vi "TreeItem.Get.vi"(8 "error in (no error)":errorcluster, 9 "Tree":T1[](array[typedef]) {"Properties"."Type" items=["K_STRING", "K_BOOL", "K_I32", "K_U32", "K_DOUBLE", "K_U64", "K_VARIANT", "K_DEPENDENTFILE", "K_DEPENDENTNODE", "K_DATASOURCENODE", "K_U16", "K_DBLARR", "K_U32ARR", "K_I32ARR", "K_STRINGARR", "K_DICTIONARY", "K_DICTIONARYARR"]}, 10 "CustomDevice BaseNode Ref":refnum<k24>, 11 "NodeIDUtil Ref":refnum<k24>) -> (0 "error out":errorcluster, 1 "Tree":T1[](array[typedef]) {"Properties"."Type" items=["K_STRING", "K_BOOL", "K_I32", "K_U32", "K_DOUBLE", "K_U64", "K_VARIANT", "K_DEPENDENTFILE", "K_DEPENDENTNODE", "K_DATASOURCENODE", "K_U16", "K_DBLARR", "K_U32ARR", "K_I32ARR", "K_STRINGARR", "K_DICTIONARY", "K_DICTIONARYARR"]}, 2 "CustomDevice BaseNode Ref out":refnum<k24>, 3 "NodeIDUtil Ref out":refnum<k24>)   [LabVIEW 2015, in "System Definition Utilities.lvlib"]
uses:
  System Definition Utilities.lvlib
  _Types/TreeItem.ctl
  _Types/TreeItem.Info.ctl
  <vilib>/NI Veristand/Custom Device API/Custom Device Channel.ctl
  <vilib>/NI Veristand/Custom Device API/Custom Device Channel Type.ctl
  <vilib>/NI Veristand/Custom Device API/Custom Device Waveform.ctl
  <vilib>/NI Veristand/Custom Device API/Custom Device Waveform DataType.ctl
  _Types/TreeItem.Property.ctl
  NationalInstruments.VeriStand.SystemStorage
  NationalInstruments.VeriStand.SystemDefinitionAPI
  <vilib>/NI Veristand/Custom Device API/Custom Device API.lvlib
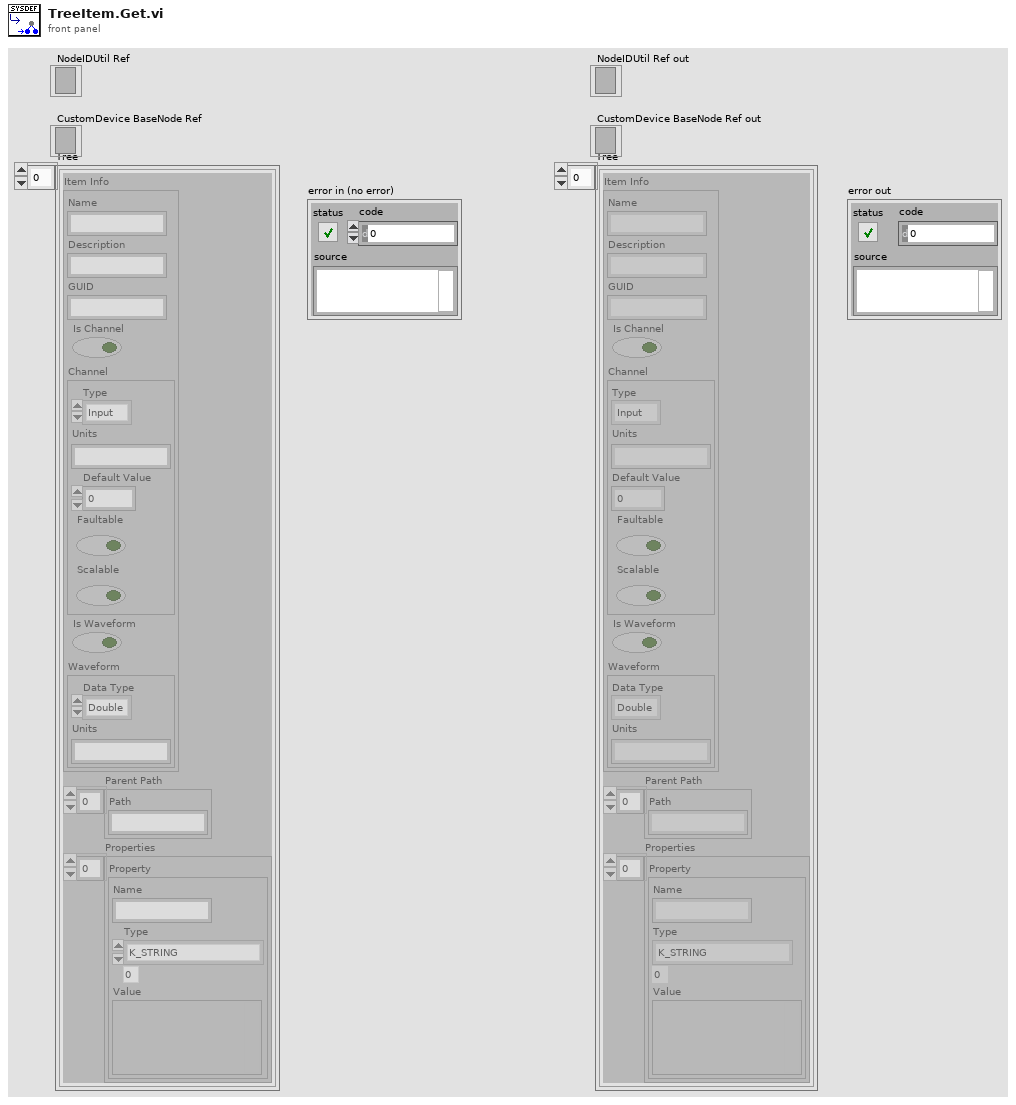
[diagram p1: front panel]
types:
  T1 = typedef "System Definition Utilities.lvlib/TreeItem.ctl" = cluster{"Item Info":T2, "Parent Path":string[], "Properties":T7[]}
  T2 = typedef "System Definition Utilities.lvlib/TreeItem.Info.ctl" = cluster{"Name":string, "Description":string, "GUID":string, "Is Channel":bool, "Channel":T3, "Is Waveform":bool, "Waveform":T5}
  T3 = typedef "Custom Device API.lvlib/Custom Device Channel.ctl" = cluster{"Type":T4, "Units":string, "Default Value":dbl, "Faultable":bool, "Scalable":bool}
  T4 = typedef "Custom Device API.lvlib/Custom Device Channel Type.ctl" = enum16{"Input", "Output"}
  T5 = typedef "Custom Device API.lvlib/Custom Device Waveform.ctl" = cluster{"Data Type":T6, "Units":string}
  T6 = typedef "Custom Device API.lvlib/Custom Device Waveform DataType.ctl" = enum16{"Double", "Complex Double"}
  T7 = typedef "System Definition Utilities.lvlib/TreeItem.Property.ctl" = cluster{"Name":string, "Type":i32, "Value":variant}
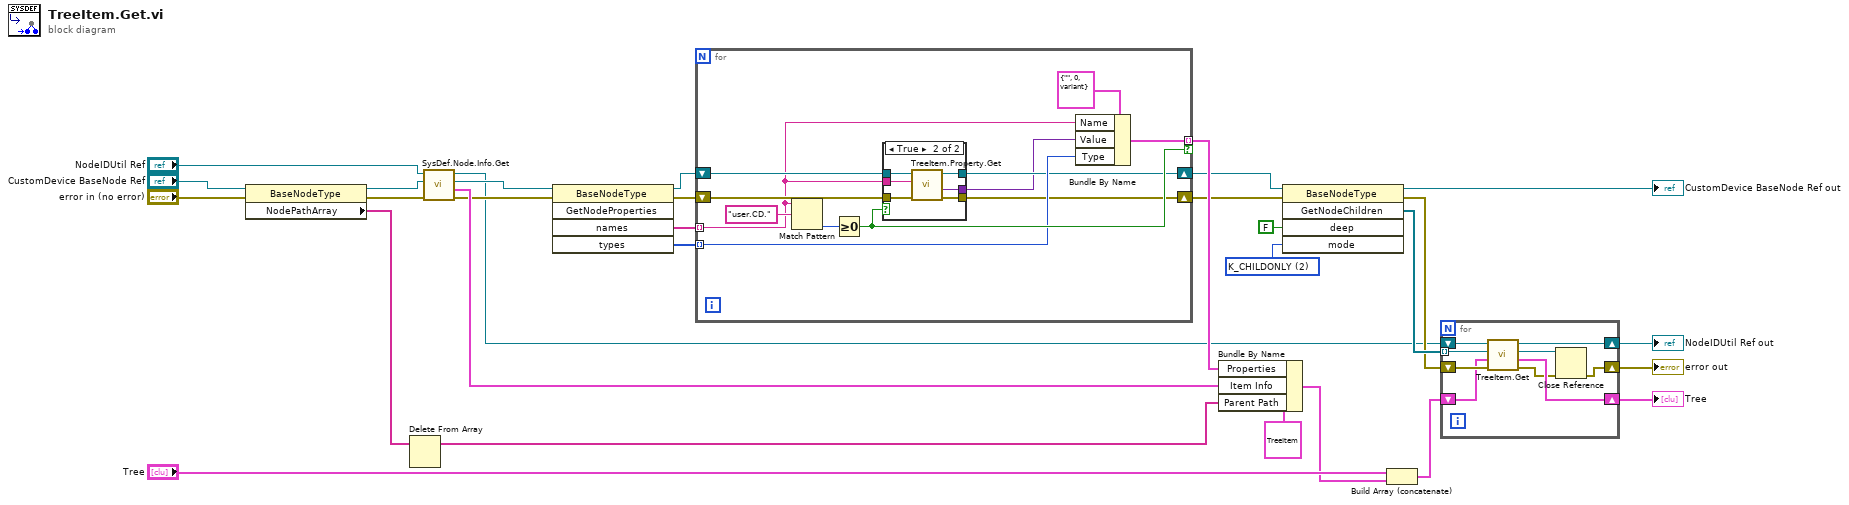
[diagram p0: block diagram]
diagram:
  w17 = 2 items=["K_BFS", "K_DFS", "K_CHILDONLY", "K_UP"] ("mode")
  n1 = property class="BaseNodeType"(reference="CustomDevice BaseNode Ref", error in="error in (no error)") -> (reference out=w3:refnum<k24>, error out=w7:errorcluster, "NodePathArray"=w5:string[])
  n2 = Delete From Array(array=w5) -> (array with subset deleted=w11:string[])  [unwired: 2 in, 1 out]
  n3 = call "SysDef.Node.Info.Get.vi"("error in (no error)"=w7, "BaseNode Ref"=w3, "NodeIDUtil Ref in"="NodeIDUtil Ref") -> ("error out"=w13:errorcluster, "Item Info"=w22:T2, "BaseNode Ref out"=w2:refnum<k24>, "NodeIDUtil Ref out"=w1:refnum<k24>)  [unwired: 5 in]
  n4 = invoke class="BaseNodeType" method="GetNodeProperties"(reference=w2, error in=w13) -> (reference out=w24:refnum<k24>, error out=w25:errorcluster, "names"=w27:string[], "types"=w26:i32[])  [unwired: 3 in, 1 out]
  n5 = for {
    tunnel: w26 -> [w35] mode=indexing
    tunnel: w27 -> [w36] mode=indexing
    shift-right: [w31] -> w20
    shift-left: w25 -> [w40]
    tunnel: [w34] -> w21 mode=indexing if=w38
    shift-right: [w33] -> w19
    shift-left: w24 -> [w39]
    n6 = Match Pattern(string=w36, regular expression="user.CD.") -> (offset past match=w41:i32)  [unwired: 1 in, 3 out]
    n7 = Greater Or Equal To 0?(x=w41) -> (x >= 0?=w38:bool)
    n8 = case shown="True" w38 {
      tunnel: w40 -> [w44 w50]
      tunnel: [w44 w49] -> w31
      tunnel: [_ w48] -> w32
      tunnel: w39 -> [w43 w47]
      tunnel: w36 -> [_ w46]
      tunnel: [w43 w45] -> w33
      frame False {
      }
      frame True {
        n9 = call "TreeItem.Property.Get.vi"("error in (no error)"=w50, "Property Name"=w46, "Basenode"=w47) -> ("error out"=w49:errorcluster, "Variant"=w48:variant, "Basenode"=w45:refnum<k24>)  [unwired: 5 in, 1 out]
      }
    }
    n10 = Bundle By Name(cluster=T7 {"Name"="", "Type"=0, "Value"=variant(string "")}, "Name"=w36, "Value"=w32, "Type"=w35) -> (w34:T7)
  }
  n11 = Bundle By Name(cluster=T1 {"Item Info"={"Name"="", "Description"="", "GUID"="", "Is Channel"=FALSE, "Channel"={"Type"=enum."Input", "Units"="", "Default Value"=0.0, "Faultable"=FALSE, "Scalable"=FALSE}, "Is Waveform"=FALSE, "Waveform"={"Data Type"=enum."Double", "Units"=""}}, "Parent Path"=[], "Properties"=[]}, "Properties"=w21, "Item Info"=w22, "Parent Path"=w11) -> (w16:T1)
  n12 = invoke class="BaseNodeType" method="GetNodeChildren"(reference=w19, error in=w20, "deep"=FALSE, "mode"=w17) -> (reference out=→"CustomDevice BaseNode Ref out":refnum<k24>, error out=w12:errorcluster, "GetNodeChildren"=w15:refnum<k24>[])  [unwired: 1 in, 2 out]
  n13 = Build Array (concatenate)("Tree", w16) -> (w14:T1[])
  n14 = for {
    tunnel: w15 -> [w56] mode=indexing
    shift-right: [w57] -> w30
    shift-left: w14 -> [w58]
    shift-right: [w52] -> w28
    shift-left: w12 -> [w59]
    shift-right: [w54] -> w10
    shift-left: w1 -> [w55]
    n15 = call "TreeItem.Get.vi"("error in (no error)"=w59, "Tree"=w58, "CustomDevice BaseNode Ref"=w56, "NodeIDUtil Ref"=w55) -> ("error out"=w53:errorcluster, "Tree"=w57:T1[], "CustomDevice BaseNode Ref out"=w51:refnum<k24>, "NodeIDUtil Ref out"=w54:refnum<k24>)  [unwired: 4 in]
    n16 = Close Reference(reference=w51, error in (no error)=w53) -> (error out=w52:errorcluster)
  }
  "Tree" <- w30
  "error out" <- w28
  "NodeIDUtil Ref out" <- w10
